vi "UDP Data Link GUID Lookup.vi"() -> ()   [LabVIEW 2015, in "UDP Data Link Shared.lvlib"]
doc: "Use this Global VI to access the GUIDs assigned to the page resources of the Custom Device."
uses:
  UDP Data Link Shared.lvlib
panel:
  in  "Status Channel Section":string="45116863-0d4e-47da-b92c-2c272c8a9276"
  in  "Chan Del Prot":string="8ea6035c-f50b-4a04-8134-22388c52d0b2"
  in  "Device":string="44d5ca09-a2d5-46d6-8443-a8ac3ee4d29c"
  in  "Status Channel":string="d537c0a0-5451-4b3d-9770-fed708507db4"
  in  "Analog Input":string="63c7125a-181b-4c57-9d03-ed07a76e0610"
  in  "Analog Input Section":string="bf23c88a-fe1c-464c-adb1-d52dd120e94d"
  in  "Task":string="0bc41655-0fbd-46a2-8ece-b4a2475f5717"
  in  "Tasks":string="3b4f2623-36ac-491d-88f5-7a83217e0976"
  in  "Custom Device":string="060ae020-2a6a-4209-a3ad-c7ce8201748e"
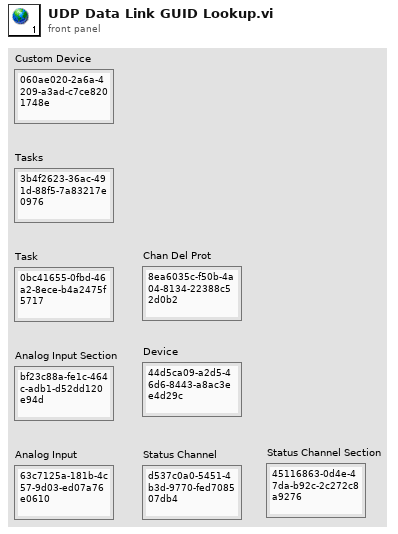
[diagram p1: front panel]
diagram:
